vi "SIM Detect Overflow or Error.vi"(0 "values":dbl[](array[numeric])) -> (1 "NaN found?":bool, 2 "Inf or NaN found?":bool, 3 "index of Inf or NaN":i32)   [LabVIEW 2010]
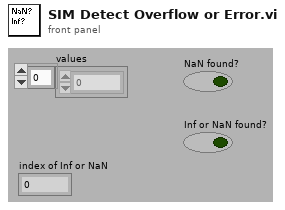
[diagram p1: front panel]
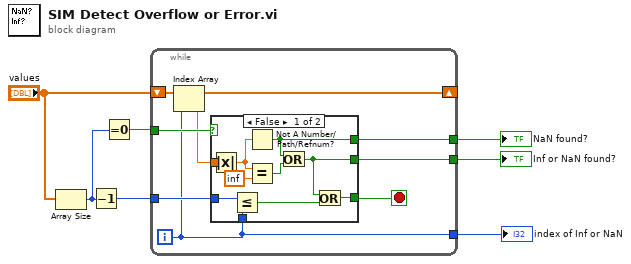
[diagram p0: block diagram]
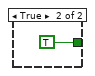
[diagram p2: hidden frame]
diagram:
  n1 = Array Size(array="values") -> (size(s)=w2:i32)
  n2 = Decrement(x=w2) -> (x-1=w3:i32)
  n3 = Equal To 0?(x=w2) -> (x = 0?=w1:bool)
  n4 = while {
    tunnel: [w15] -> w6
    tunnel: [w14] -> w7
    tunnel: [w10] -> w4
    tunnel: w3 -> [w13]
    tunnel: w1 -> [w11]
    shift-right: [w8] -> _
    shift-left: "values" -> [w8]
    i -> [w10]
    stop <- w12 stop-if-true
    n5 = Index Array(array=w8, index=w10) -> (element=w9:dbl)
    n6 = case shown="False" w11 {
      tunnel: [w25 _] -> w15
      tunnel: [w24 _] -> w14
      tunnel: w10 -> [w23 _]
      tunnel: w13 -> [w22 _]
      tunnel: w9 -> [w21 _]
      tunnel: [w20 TRUE] -> w12
      frame False {
        n7 = Absolute Value(x=w21) -> (abs(x)=w16:dbl)
        n8 = Less Or Equal?(x=w22, y=w23) -> (x <= y?=w19:bool)
        n9 = Not A Number/Path/Refnum?(number/path/refnum=w16) -> (NaN/Path/Refnum?=w24:bool)
        n10 = Equal?(x=w16, y=inf) -> (x = y?=w18:bool)
        n11 = Or(x=w24, y=w18) -> (x .or. y?=w25:bool)
        n12 = Or(x=w25, y=w19) -> (x .or. y?=w20:bool)
      }
      frame True {
      }
    }
  }
  "NaN found?" <- w7
  "Inf or NaN found?" <- w6
  "index of Inf or NaN" <- w4
